vi "ReadFromSIngelFile.vi"(8 "error in (no error)":errorcluster, 10 "FilePath":path, 11 "RawData":T1(array[cluster])) -> (0 "error out":errorcluster, 2 "XYData":cluster{"X":dbl[], "Y":dbl[]}[](array[cluster]), 3 "RawDataOut":T1(array[cluster]))   [LabVIEW 2012]
doc: "读取单个文件的数据；\nName：蒋松\nEmail：jiangsong@outlook.com"
uses:
  <vilib>/Utility/file.llb/Read From Spreadsheet File (DBL).vi
panel:
  # "VI INPUTS"
  # "VI OUTPUTS"
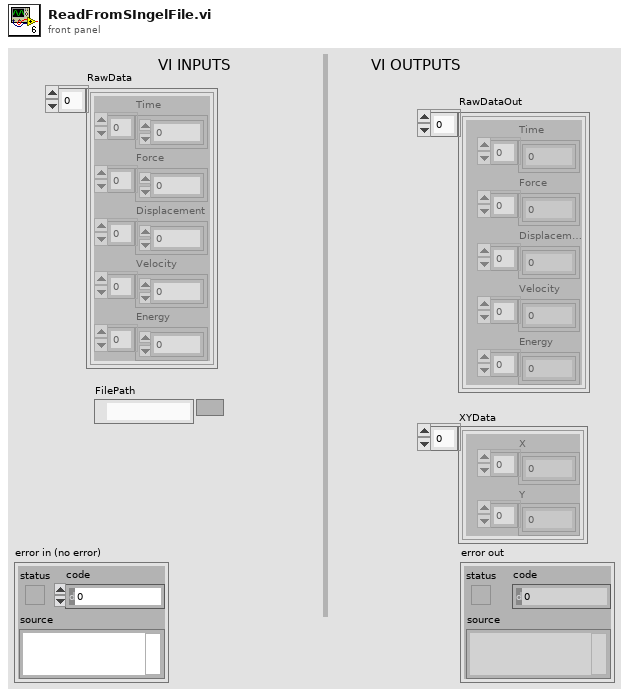
[diagram p1: front panel]
types:
  T1 = cluster{"Time":dbl[], "Force":dbl[], "Displacement":dbl[], "Velocity":dbl[], "Energy":dbl[]}[]
  T2 = cluster{"Time":dbl[], "Force":dbl[], "Displacement":dbl[], "Velocity":dbl[], "Energy":dbl[]}
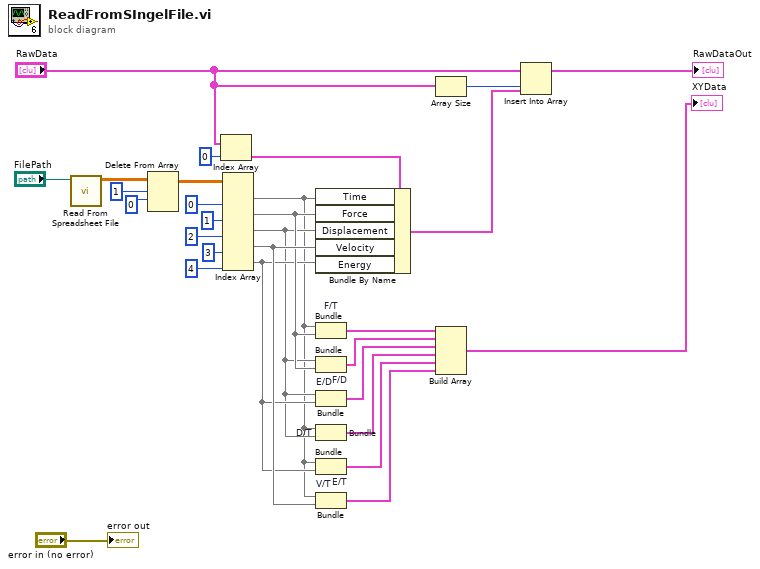
[diagram p0: block diagram]
diagram:
  n1 = call-poly <vilib>:"Read From Spreadsheet File.vi"("file path (dialog if empty)"="FilePath") -> ("all rows"=w24:dbl[][])  [unwired: 6 in, 4 out]
  n2 = Delete From Array(array=w24, length=1, index (row)=0) -> (array with subset deleted=w23:dbl[][])  [unwired: 1 in, 1 out]
  n3 = Index Array(array="RawData", index=0) -> (element=w17:T2)
  n4 = Index Array(array=w23, index (col) #1=0 ("index (row)"), index (col) #2=1 ("index (row)"), index (col) #3=2 ("index (row)"), index (col) #4=3 ("index (row)"), index (col) #5=4 ("index (row)")) -> (element #1=w3:dbl[], element #2=w12:dbl[], element #3=w10:dbl[], element #4=w13:dbl[], element #5=w11:dbl[])  [unwired: 5 in]
  n5 = Bundle By Name(cluster=w17, "Time"=w3, "Force"=w12, "Displacement"=w10, "Velocity"=w13, "Energy"=w11) -> (w16:T2)
  n6 = Bundle "F/T"("all rows"=w3, "all rows"=w12) -> (w9:cluster{"all rows":dbl[], "all rows":dbl[]})  [unwired: 1 in]
  n7 = Bundle "F/D"("all rows"=w10, "all rows"=w12) -> (w8:cluster{"all rows":dbl[], "all rows":dbl[]})  [unwired: 1 in]
  n8 = Bundle "E/D"("all rows"=w10, "all rows"=w11) -> (w7:cluster{"all rows":dbl[], "all rows":dbl[]})  [unwired: 1 in]
  n9 = Bundle "D/T"("all rows"=w3, "all rows"=w10) -> (w6:cluster{"all rows":dbl[], "all rows":dbl[]})  [unwired: 1 in]
  n10 = Bundle "E/T"("all rows"=w3, "all rows"=w11) -> (w5:cluster{"all rows":dbl[], "all rows":dbl[]})  [unwired: 1 in]
  n11 = Bundle "V/T"("all rows"=w3, "all rows"=w13) -> (w4:cluster{"all rows":dbl[], "all rows":dbl[]})  [unwired: 1 in]
  n12 = Array Size(array="RawData") -> (size(s)=w15:i32)
  n13 = Build Array(w9, w8, w7, w6, w5, w4) -> (→"XYData":cluster{"all rows":dbl[], "all rows":dbl[]}[])
  n14 = Insert Into Array(array="RawData", index=w15, new element=w16) -> (→"RawDataOut":T1)
  "error out" <- "error in (no error)"
